vi "Config Parser Test.vi"() -> ()   [LabVIEW 2018]
uses:
  Interfaces/File Parser Interface.lvlibp/Ctls/Protocol Type.ctl
  Ctls/FRM Data - BML.ctl
  Ctls/OM - BML.ctl
  Ctls/Burst Length.ctl
  Ctls/RW Options.ctl
  Ctls/Frame Data - SPI_3W.ctl
  Ctls/Protocol Type.ctl
  Interfaces/File Parser Interface.lvlibp/Interfaces/File Parser Interface/File Parser Interface.lvclass
  Interfaces/File Parser Interface.lvlibp
panel:
  in  "Protocol Type":T1
  out "Array 2":T2[](array[typedef]) {"Addr" format="%x"; "Data" format="%x"}
  out "Array":T4[](array[typedef]) {"Start_Addr" format="%x"; "Data" format="%x"}
  out "error out":errorcluster
  out "Protocol Type out":T7
  in  "Config File":path
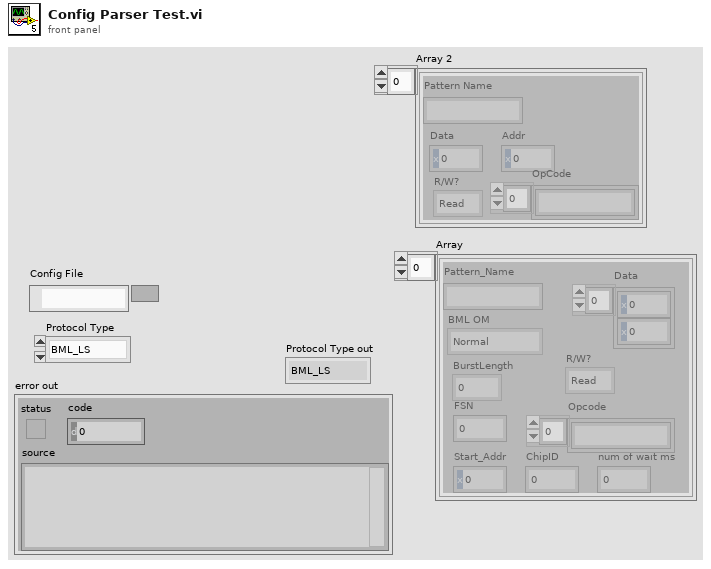
[diagram p1: front panel]
types:
  T1 = typedef "Protocol Type.ctl" = enum16{"BML_LS", "BML_HS", "SPI_3W", "SPI_4W"}
  T2 = typedef "Frame Data - SPI_3W.ctl" = cluster{"Pattern Name":string, "Data":u16, "Addr":u16, "OpCode":string[], "R/W?":T3}
  T3 = typedef "RW Options.ctl" = enum16{"Read", "Write", "R/W"}
  T4 = typedef "FRM Data - BML.ctl" = cluster{"Pattern_Name":string, "Data":u8[], "Start_Addr":u16, "ChipID":u8, "num of wait ms":i8, "Opcode":string[], "BML OM":T5, "BurstLength":T6, "FSN":u8, "R/W?":T3}
  T5 = typedef "OM - BML.ctl" = enum16{"Normal", "ImmeEffect", "InitSlaveID", "LoadData"}
  T6 = typedef "Burst Length.ctl" = enum8{"0", "2", "3", "4", "5", "8", "16", "32"}
  T7 = typedef "File Parser Interface.lvlibp/Protocol Type.ctl" = enum16{"BML_LS", "BML_HS", "SPI_3W", "SPI_4W"}
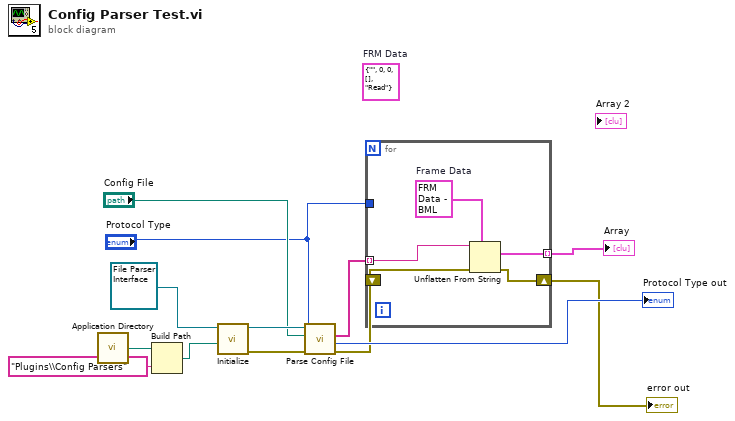
[diagram p0: block diagram]
diagram:
  (unwired) T2 {"Pattern Name"="", "Data"=0, "Addr"=0, "OpCode"=[], "R/W?"=enum."Read"}  # FRM Data
  n1 = call <vilib>:"Application Directory.vi"() -> ("Application Directory"=w13:path)
  n2 = Build Path(base path=w13, name or relative path="Plugins\\Config Parsers") -> (appended path=w11:path)
  n3 = call-dynamic "Initialize.vi"("Plugin Folder"=w11, "File Parser Interface in"=refnum<class "File Parser Interface.lvclass"> refnum ("File Parser Interface.lvlibp:File Parser Interface.lvclass")) -> ("error out"=w6:errorcluster, "File Parser Interface out"=w10:refnum<class "File Parser Interface.lvclass">)  [unwired: 8 in]
  n4 = call "Parse Config File.vi"("error in (no error)"=w6, "Protocol Type in"="Protocol Type", "Config File"="Config File", "File Parser Interface in"=w10) -> ("error out"=w5:errorcluster, "Protocol Type out"=→"Protocol Type out":T7, "Config Array"=w7:string[])  [unwired: 4 in, 1 out]
  n5 = for {
    tunnel: w7 -> [w18] mode=indexing
    tunnel: "Protocol Type" -> [_]
    tunnel: [w17] -> w1 mode=indexing
    shift-right: [w15] -> w4
    shift-left: w5 -> [w16]
    w14 = T4 {"Pattern_Name"="", "Data"=[], "Start_Addr"=0, "ChipID"=1, "num of wait ms"=0, "Opcode"=[], "BML OM"=enum."Normal", "BurstLength"=enum."0", "FSN"=0, "R/W?"=enum."Read"}  # Frame Data
    n6 = Unflatten From String(type=w14, binary string=w18, error in (no error)=w16) -> (value=w17:T4, error out=w15:errorcluster)  [unwired: 2 in, 1 out]
  }
  "error out" <- w4
  "Array" <- w1
